vi "build load configuration commands.vi"(8 "error in (no error)":errorcluster, 10 "configuration name":string, 11 "Device name":string) -> (0 "error out":errorcluster, 2 "load configuration info":T1, 3 "loadconfigCommands":string)   [LabVIEW 2020]
uses:
  load configuration_typdef.ctl
  Preset Query Enum.ctl
panel:
  out "data":string[][](array[string])
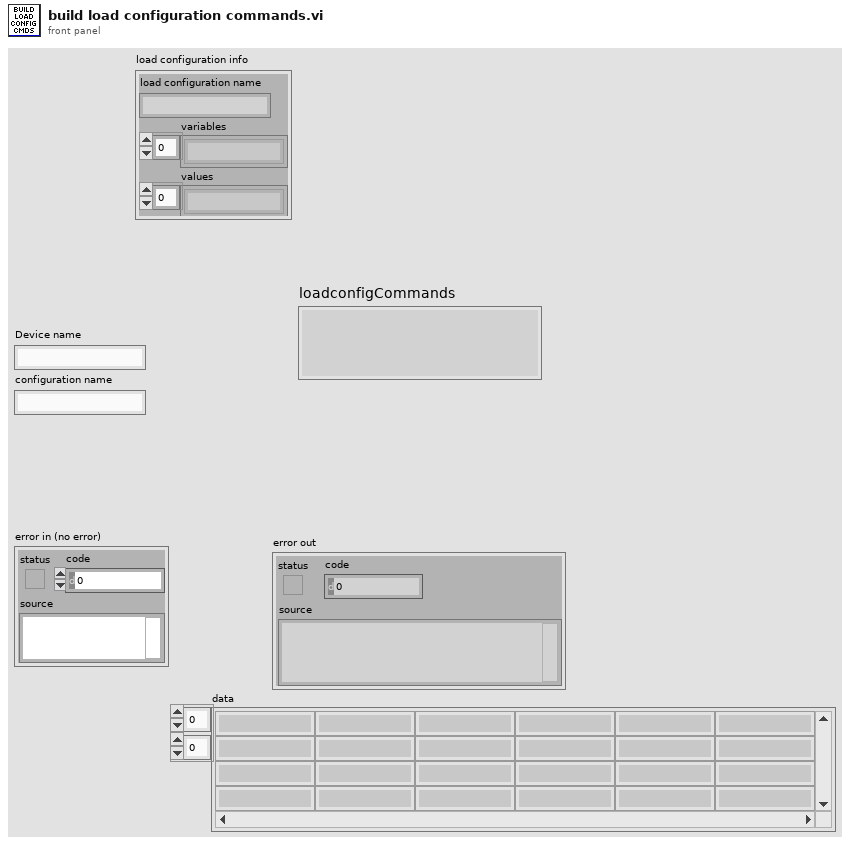
[diagram p1: front panel]
types:
  T1 = typedef "load configuration_typdef.ctl" = cluster{"load configuration name":string, "variables":string[], "values":string[]}
  T2 = typedef "Preset Query Enum.ctl" = enum16{"Get Locations", "Get all IPs and MACs", "Get classes", "Get expt variables to set at scanstart for particular device", "Get expt devices and variables with start values", "Get expt devices and variables (with data to get)", "Get expt devices with data to get", "Get Expt devices and GUIs", "Get all devices basic properties", "Get Virtual Devices Core Info", "Get Expt names", "Get experiment basic properties", "Get experiment alarm variables", "Get MC Ports", "Get device network comm port", "Get devicetype lvclass path", "Get basic device properties", "Get Init Order", "Get all setable variables of a device", "Get device variable aliases", "Get force values of all settable variables", "Get all variables of a devicetype", "Get all variables of a device", "Get plotter details", "Get Saved Scans", "Get Scan Info", "GetGeneralGUIs", "Get expt for plotter", "Get plotter IDs from expt", "Get all devices", "Get all Virtual Devices", "Get all aliases", "Get variable and device info for Virtual Device", "GetItemLocatorIP", "Get IPs for GUIs", "Get DeviceType from Device", "GetLocalPortRange", "GetDevicePresetVariables", "Get Device Configuration", "GetAllPresetNames", "GetAllConfigurationNames", "GetPresetDeviceNames", "GetDeviceAliases", "GetDevicesOfClass"}
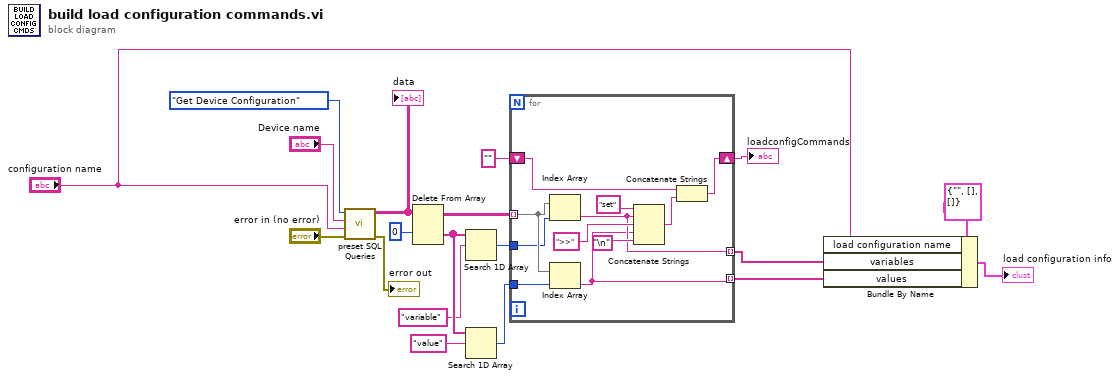
[diagram p0: block diagram]
diagram:
  n1 = call "preset SQL Queries.vi"("error in (no error)"="error in (no error)", "Expt name / MCIP/ Variable/Preset Name"="configuration name", "Device/Devicetype name\n/Plotter.id/ScanName#"="Device name", "Preset Query"=Preset_Query_Enum."Get Device Configuration") -> ("error out"=→"error out":errorcluster, "data"=w5:string[][])  [unwired: 5 in, 1 out]
  "data" <- w5
  n2 = Delete From Array(array=w5, index (row)=0) -> (deleted portion=w10:string[], array with subset deleted=w7:string[][])  [unwired: 2 in]
  n3 = Search 1D Array(1D array=w10, element="variable") -> (index of element=w11:i32)  [unwired: 1 in]
  n4 = Search 1D Array(1D array=w10, element="value") -> (index of element=w8:i32)  [unwired: 1 in]
  n5 = for {
    tunnel: w7 -> [w29] mode=indexing
    tunnel: w8 -> [w30]
    tunnel: w11 -> [w28]
    shift-right: [w23] -> w13
    shift-left: "" -> [w22]
    tunnel: [w21] -> w18 mode=indexing
    tunnel: [w20] -> w19 mode=indexing
    n6 = Index Array(array=w29, index=w28) -> (element=w21:string)
    n7 = Index Array(array=w29, index=w30) -> (element=w20:string)
    n8 = Concatenate Strings("set", w21, ">>" ("string"), w20, "\n") -> (w24:string)
    n9 = Concatenate Strings(w22, w24) -> (w23:string)
  }
  "loadconfigCommands" <- w13
  n10 = Bundle By Name(cluster=T1 {"load configuration name"="", "variables"=[], "values"=[]} ("load configuration info"), "load configuration name"="configuration name", "variables"=w18, "values"=w19) -> (→"load configuration info":T1)
